vi "run.vi"(8 "error in (no error)":errorcluster, 11 "GenericPlugin in":refnum<class "ComponentTemplate.lvclass">) -> (0 "error out":errorcluster, 3 "GenericPlugin out":refnum<class "ComponentTemplate.lvclass">)   [LabVIEW 2010, in "ComponentTemplate.lvclass"]
uses:
  ComponentTemplate.lvclass
  common/classes/GenericComponent/GenericComponent/GenericComponent.lvclass
  common/classes/ErrorController/ErrorController/ErrorController.lvclass
panel:
  in  "Tab Control":enum32{"User", "Debug", "About"}(tab)
  in  "return to origin?":bool=TRUE
  out "finished?":bool
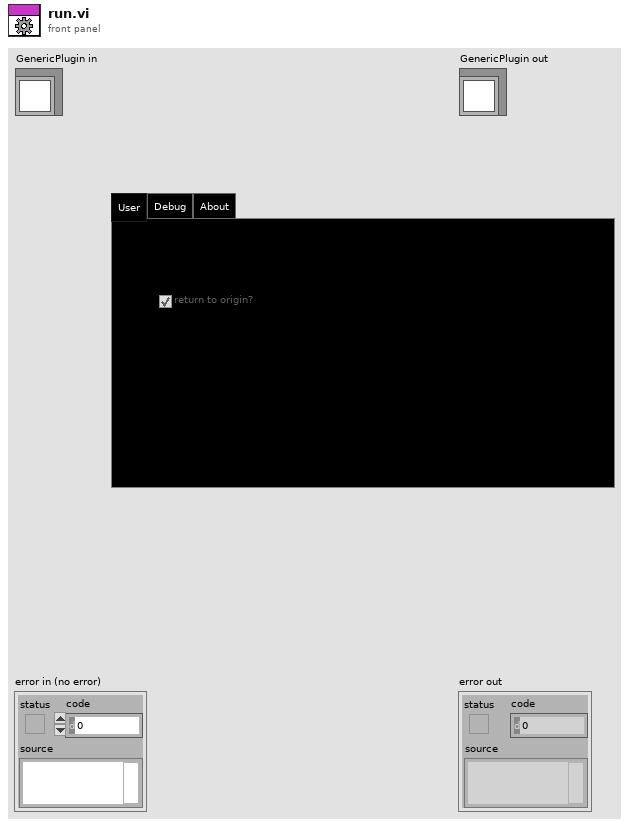
[diagram p1: front panel]
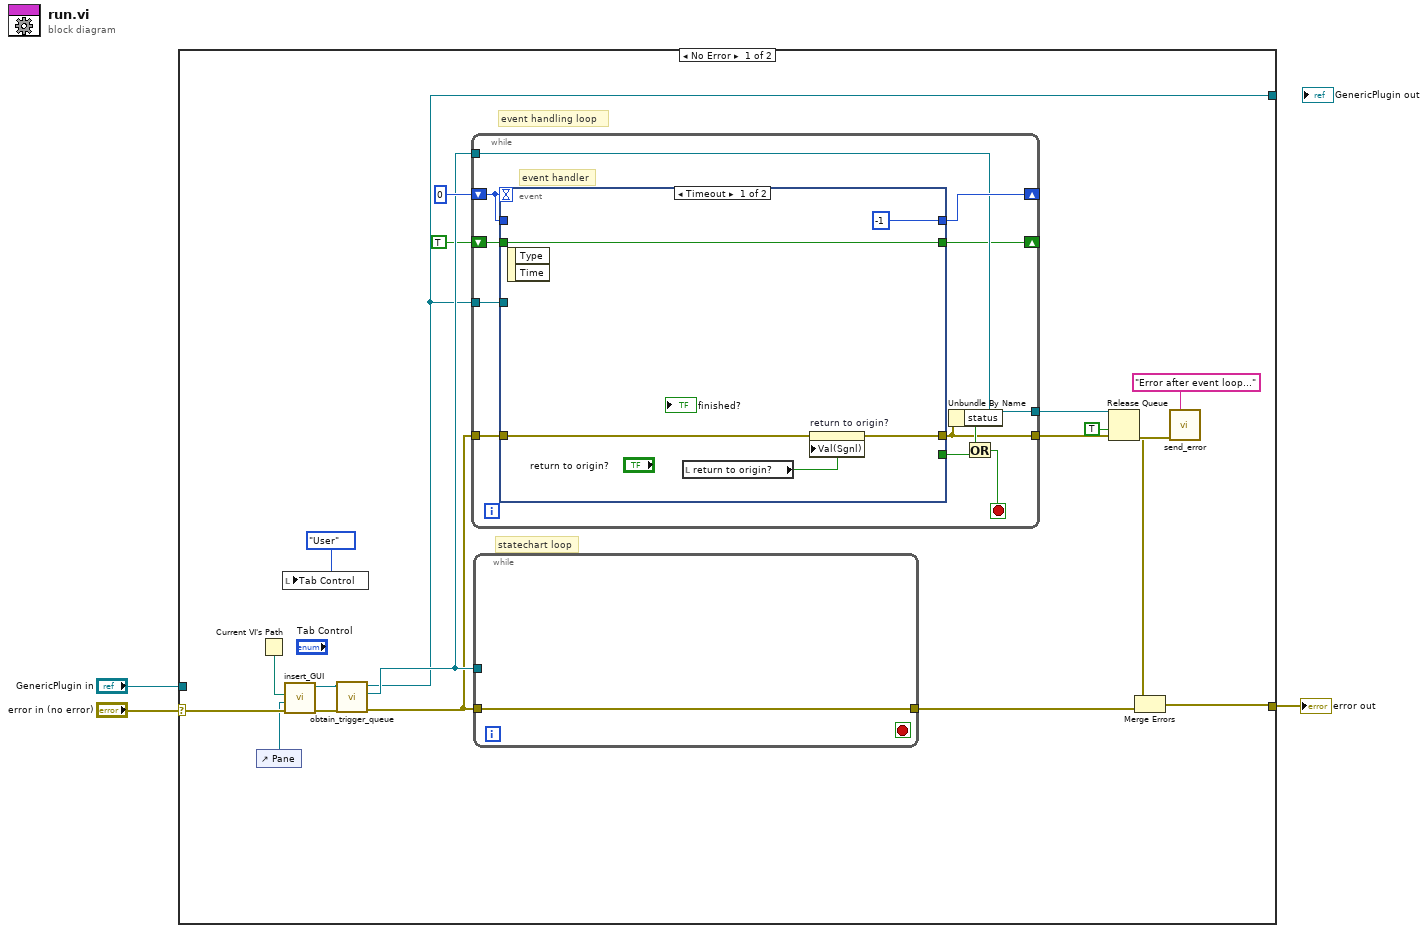
[diagram p0: block diagram]
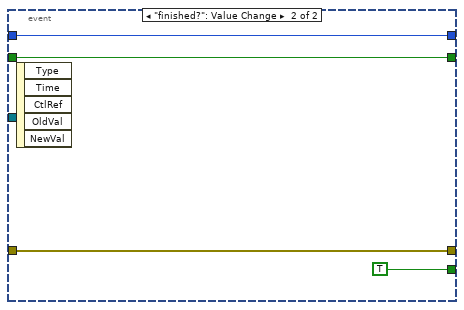
[diagram p2: hidden frame]
diagram:
  n1 = case shown="No Error" "error in (no error)" {
    selector: "error in (no error)" -> [w21 w44]
    tunnel: [w7 w44] -> w2
    tunnel: "GenericPlugin in" -> [_ w45]
    tunnel: [w6 w45] -> _
    frame No Error {
      # "event handling loop"
      # "statechart loop"
      n2 = control-ref of="Pane"() -> (w18:refnum<vi>)
      n3 = Current VI's Path() -> (path=w17:path)
      n4 = local write "Tab Control"(enum32{"User", "Debug", "About"}."User" ("Tab Control")) -> ()
      n5 = call-dynamic "insert_GUI.vi"("error in (no error)"=w21, "Pane"=w18, "VI path"=w17) -> ("error out"=w20:errorcluster, "GenericComponent out"=w19:refnum<class "GenericComponent.lvclass">)  [unwired: 7 in]
      n6 = call-dynamic "obtain_trigger_queue.vi"("error in (no error)"=w20, "GenericPlugin in"=w19) -> ("error out"=w15:errorcluster, "trigger queue"=w16:refnum<queue>, "GenericPlugin out"=w6:refnum<class "GenericComponent.lvclass">)  [unwired: 7 in]
      n7 = while {
        shift-right: [w33] -> _
        shift-left: 0 -> [w34]
        tunnel: w6 -> [w32]
        tunnel: w16 -> [w26]
        tunnel: w15 -> [w31]
        tunnel: [w27] -> w11
        tunnel: [w26] -> w12
        shift-right: [w24] -> _
        shift-left: TRUE -> [w25]
        stop <- w29 stop-if-true
        # "event handler"
        n8 = event shown="[0] Timeout" {
          selector: _ -> [_ _]
          dyn-events: _ -> [_ _]
          timeout: w34 -> [_ _]
          tunnel: [-1 w43] -> w33
          tunnel: w34 -> [_ w43]
          tunnel: w32 -> [_ _]
          tunnel: w31 -> [w37 w41]
          tunnel: [w36 w41] -> w27
          tunnel: [_ TRUE] -> w30
          tunnel: w25 -> [w35 w40]
          tunnel: [w35 w40] -> w24
          event Timeout {
            n9 = event-data() -> ()  [unwired: 1 in, 2 out]
            n10 = local read "return to origin?"() -> (w38:bool)
            n11 = property on="return to origin?" class="Bool (strict)"(error in=w37, "Val(Sgnl)"=w38) -> (error out=w36:errorcluster)  [unwired: 1 in, 1 out]
          }
          event "finished?": Value Change {
            n12 = event-data() -> ()  [unwired: 1 in, 5 out]
          }
        }
        n13 = Unbundle By Name(w27) -> ("status"=w28:bool)
        n14 = Or(x=w28, y=w30) -> (x .or. y?=w29:bool)
      }
      n15 = while {
        tunnel: w16 -> [_]
        tunnel: w15 -> [w23]
        tunnel: [w23] -> w8
        stop <- _ stop-if-true
      }
      n16 = Release Queue(queue=w12, force destroy? (F)=TRUE, error in (no error)=w11) -> (error out=w14:errorcluster)  [unwired: 2 out]
      n17 = call "send_error.vi"("additional message"="Error after event loop...", "error in (no error)"=w14) -> ("error out"=w9:errorcluster)  [unwired: 9 in]
      n18 = Merge Errors(w9, w8) -> (w7:errorcluster)
    }
    frame Error {
    }
  }
  "error out" <- w2
